vi "实验5_2.vi"() -> ()   [LabVIEW 2018]
panel:
  out "String":string
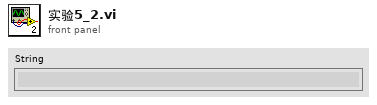
[diagram p1: front panel]
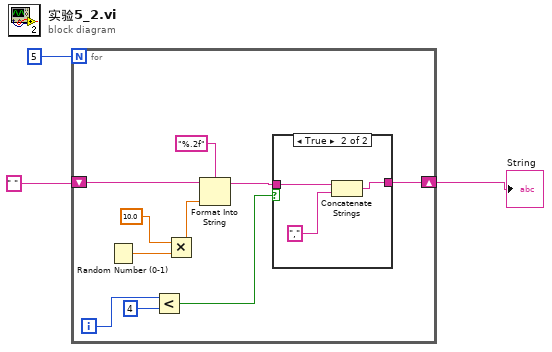
[diagram p0: block diagram]
diagram:
  n1 = for {
    N: 5 -> [_]
    shift-right: [w4] -> w1
    shift-left: " " -> [w6]
    i -> [w12]
    n2 = Random Number (0-1)() -> (number: 0 to 1=w10:dbl)
    n3 = Less?(x=w12, y=4) -> (x < y?=w8:bool)
    n4 = Multiply(x=10.0, y=w10) -> (x*y=w5:dbl)
    n5 = Format Into String(format string="%.2f", initial string=w6, w5) -> (resulting string=w7:string)  [unwired: 1 in, 1 out]
    n6 = case shown="True" w8 {
      tunnel: w7 -> [w14 w16]
      tunnel: [w14 w15] -> w4
      frame False {
      }
      frame True {
        n7 = Concatenate Strings(w16, ",") -> (w15:string)
      }
    }
  }
  "String" <- w1
